vi "Close.vi"(8 "error in (no error)":errorcluster, 11 "FPGA Interface in":refnum<class "FPGA Interface.lvclass">) -> (0 "error out":errorcluster)   [LabVIEW 2020, in "BCI-1553 API.lvlib" / "FPGA Interface.lvlib" / "FPGA Interface.lvclass"]
doc: "Ends the FPGA session that is supporting the communication with the BCI-1553 modules."
uses:
  FPGA Interface.lvclass
  FPGA Interface.lvclass/FPGA Interface.ctl
  <vilib>/FPGAPlugInAG/Dynamic/niLvFpga_Close_Dynamic.vi
  <vilib>/rvi/interface/nirviCloseFPGA/nirviCloseFPGA.xnode
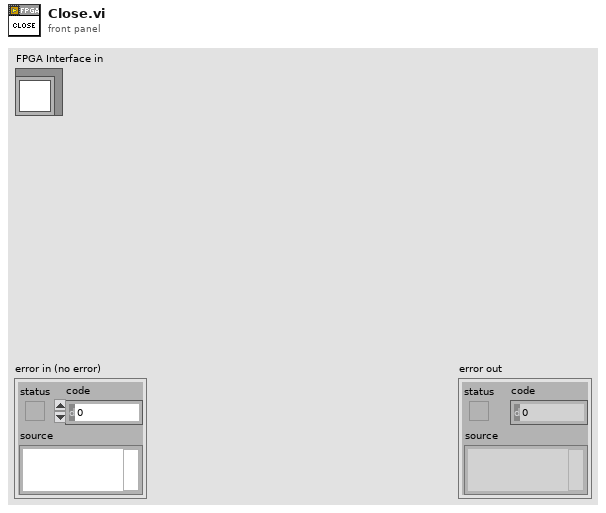
[diagram p1: front panel]
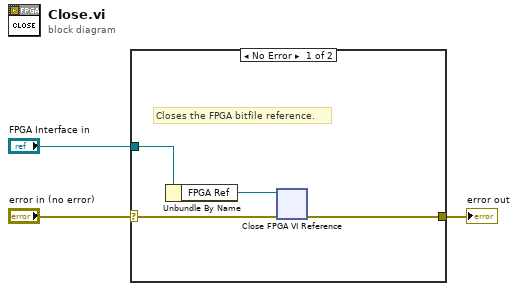
[diagram p0: block diagram]
diagram:
  n1 = case shown="No Error" "error in (no error)" {
    selector: "error in (no error)" -> [w5 w8]
    tunnel: [w4 w8] -> w2
    tunnel: "FPGA Interface in" -> [w7 _]
    frame No Error {
      # "Closes the FPGA bitfile reference."
      n2 = Unbundle By Name(w7) -> ("FPGA Ref"=w6:refnum<k20>)
      n3 = xnode "Close FPGA VI Reference"("FPGA VI Reference In"=w6, "error in"=w5) -> ("error out"=w4:errorcluster)
    }
    frame Error {
    }
  }
  "error out" <- w2
